vi "Control Coefficients Updating for Adaptive Filter.vi"() -> ()   [LabVIEW 2023]
doc: "This example demonstrates how to use the AFT Filter Signal VI and the AFT Update Coefficients VI together. By using these two VIs, you can specify whether and when to update the coefficients of an adaptive filter.\n\nWhen you run this VI, the coefficients of the adaptive filter begin to converge to the coefficients of the unknown system. If you click the <b>Update Coefficients</b> button, this example applies only linear filtering to the input signal. Therefore, the coefficients stop updating. Click this button again to resume updating the coefficients.\n\nThis example uses an FIR LMS adaptive filter to identify the impulse response of an unknown system. A lowpass FIR filter simulates the unknown system. The input to both this system and the adaptive filter is Gaussian white noise. The output of this system is the reference of the adaptive filter.\n\nRefer to the Adaptive Channel Equalization example in the <b>Applications</b> folder for information about using the AFT Filter Signal VI and the AFT Update Coefficients VI in adaptive channel equalization applications."
uses:
  <vilib>/addons/Adaptive Filters/Create/AFT Create FIR LMS (Real).vi
  <vilib>/addons/Adaptive Filters/Processing/AFT Filter Signal (Real, PtByPt).vi
  <vilib>/addons/Adaptive Filters/Processing/AFT Update Coefficients (Real, PtByPt).vi
  <vilib>/addons/Adaptive Filters/Analysis/AFT Get Coefficients (FIR, Real).vi
  <vilib>/addons/Adaptive Filters/NI_AdaptiveFilter.lvlib
panel:
  out "Error Signal":dbl(graph)
  in  "Reset":bool
  in  "Update Coefficients":bool=TRUE
  in  "Step Size":dbl=0.002 min=1e-16 step=0.001
  in  "Filter Length":i32=25 min=2
  out "Coefficients":dbl[][](graph)
  in  "Stop":bool
  # "Select Help>>Show Context Help and move the cursor over the VI icon of this example for more information."
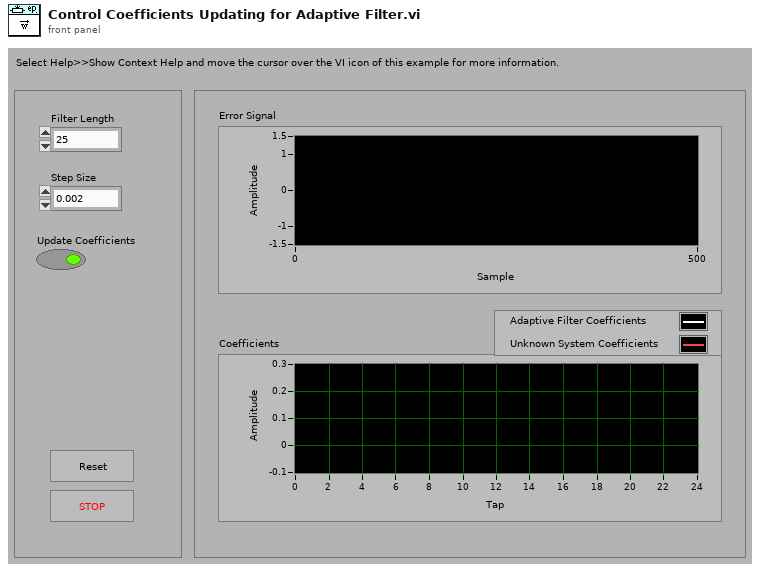
[diagram p1: front panel]
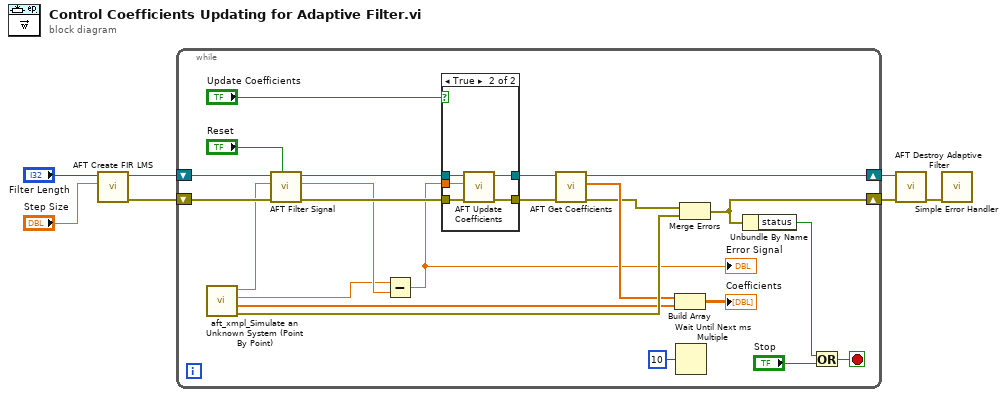
[diagram p0: block diagram]
diagram:
  n1 = call-poly <vilib>:"AFT Create FIR LMS.vi"("step size"="Step Size", "filter length"="Filter Length") -> ("error out"=w5:errorcluster, "adaptive filter out"=w6:refnum<k20>)  [unwired: 2 in, 6 out]
  n2 = while {
    shift-right: [w29] -> w4
    shift-left: w6 -> [w25]
    shift-right: [w11] -> w3
    shift-left: w5 -> [w24]
    stop <- w9 stop-if-true
    n3 = call "aft_xmpl_Simulate an Unknown System (Point By Point).vi"() -> ("error out"=w30:errorcluster, "unknown system coefficients"=w13:dbl[], "response signal"=w14:dbl, "stimulus signal"=w15:dbl)  [unwired: 1 in, 7 out]
    n4 = call-poly <vilib>:"AFT Filter Signal.vi"("reset? (F)"="Reset", "error in (no error)"=w24, "x(n)"=w15, "adaptive filter in"=w25) -> ("error out"=w21:errorcluster, "y(n)"=w17:dbl, "adaptive filter out"=w23:refnum<k20>)  [unwired: 5 out]
    n5 = Subtract(x=w14, y=w17) -> (x-y=w16:dbl)
    "Error Signal" <- w16
    n6 = case shown="True" "Update Coefficients" {
      tunnel: w23 -> [w32 w37]
      tunnel: [w32 w36] -> w22
      tunnel: w21 -> [w31 w35]
      tunnel: [w31 w34] -> w20
      tunnel: w16 -> [_ w33]
      frame False {
      }
      frame True {
        n7 = call-poly <vilib>:"AFT Update Coefficients.vi"("error in (no error)"=w35, "e(n)"=w33, "adaptive filter in"=w37) -> ("error out"=w34:errorcluster, "adaptive filter out"=w36:refnum<k20>)  [unwired: 1 in, 6 out]
      }
    }
    n8 = call-poly <vilib>:"AFT Get Coefficients.vi"("error in (no error)"=w20, "adaptive filter in"=w22) -> ("error out"=w12:errorcluster, "coefficients"=w28:dbl[], "adaptive filter out"=w29:refnum<k20>)  [unwired: 7 out]
    n9 = Build Array(w28, w13) -> (→"Coefficients":dbl[][])
    n10 = Wait Until Next ms Multiple(millisecond multiple=u32 10) -> ()  [unwired: 1 out]
    n11 = Merge Errors(w12, w30) -> (w11:errorcluster)
    n12 = Unbundle By Name(w11) -> ("status"=w8:bool)
    n13 = Or(x=w8, y="Stop") -> (x .or. y?=w9:bool)
  }
  n14 = call <vilib>:"AFT Destroy Adaptive Filter.vi"("error in (no error)"=w3, "adaptive filter in"=w4) -> ("error out"=w1:errorcluster)  [unwired: 9 out]
  n15 = call <vilib>:"Simple Error Handler.vi"("error in (no error)"=w1) -> ()  [unwired: 1 in, 8 out]
